vi "single_window_time_all_in_one.vi"(8 "Error In":errorcluster, 9 "Ship data?":bool, 10 "controls":T1={"window duration"=1.0, "width"=5, "crossing level"=0.0, "threshold"=0.25, "Sec"=1.0, "start time"=0.0, "correction thresholds"=[25, 20, 20, 30]} {"start time" format="%#_13g"; "Sec" format="%0.2f"; "threshold" format="%0.2f"; "crossing level" format="%#_13g"; "width" min=3; "window duration" format="%0.2f"}, 11 "waveform in":waveform(dbl)) -> (0 "Error out":errorcluster, 3 "time data cluster":T2 {"variance  of w/a ratio" format="%0.2f"; "sd  of w/a ratio" format="%0.2f"; "mean of w/a ratio" format="%0.2f"})   [LabVIEW 2020]
uses:
  <vilib>/Waveform/WDTOps.llb/WDT Get Waveform Subset DBL.vi
  <vilib>/Analysis/NI_AALBase.lvlib
panel:
  out "XY Graph":T3(graph)
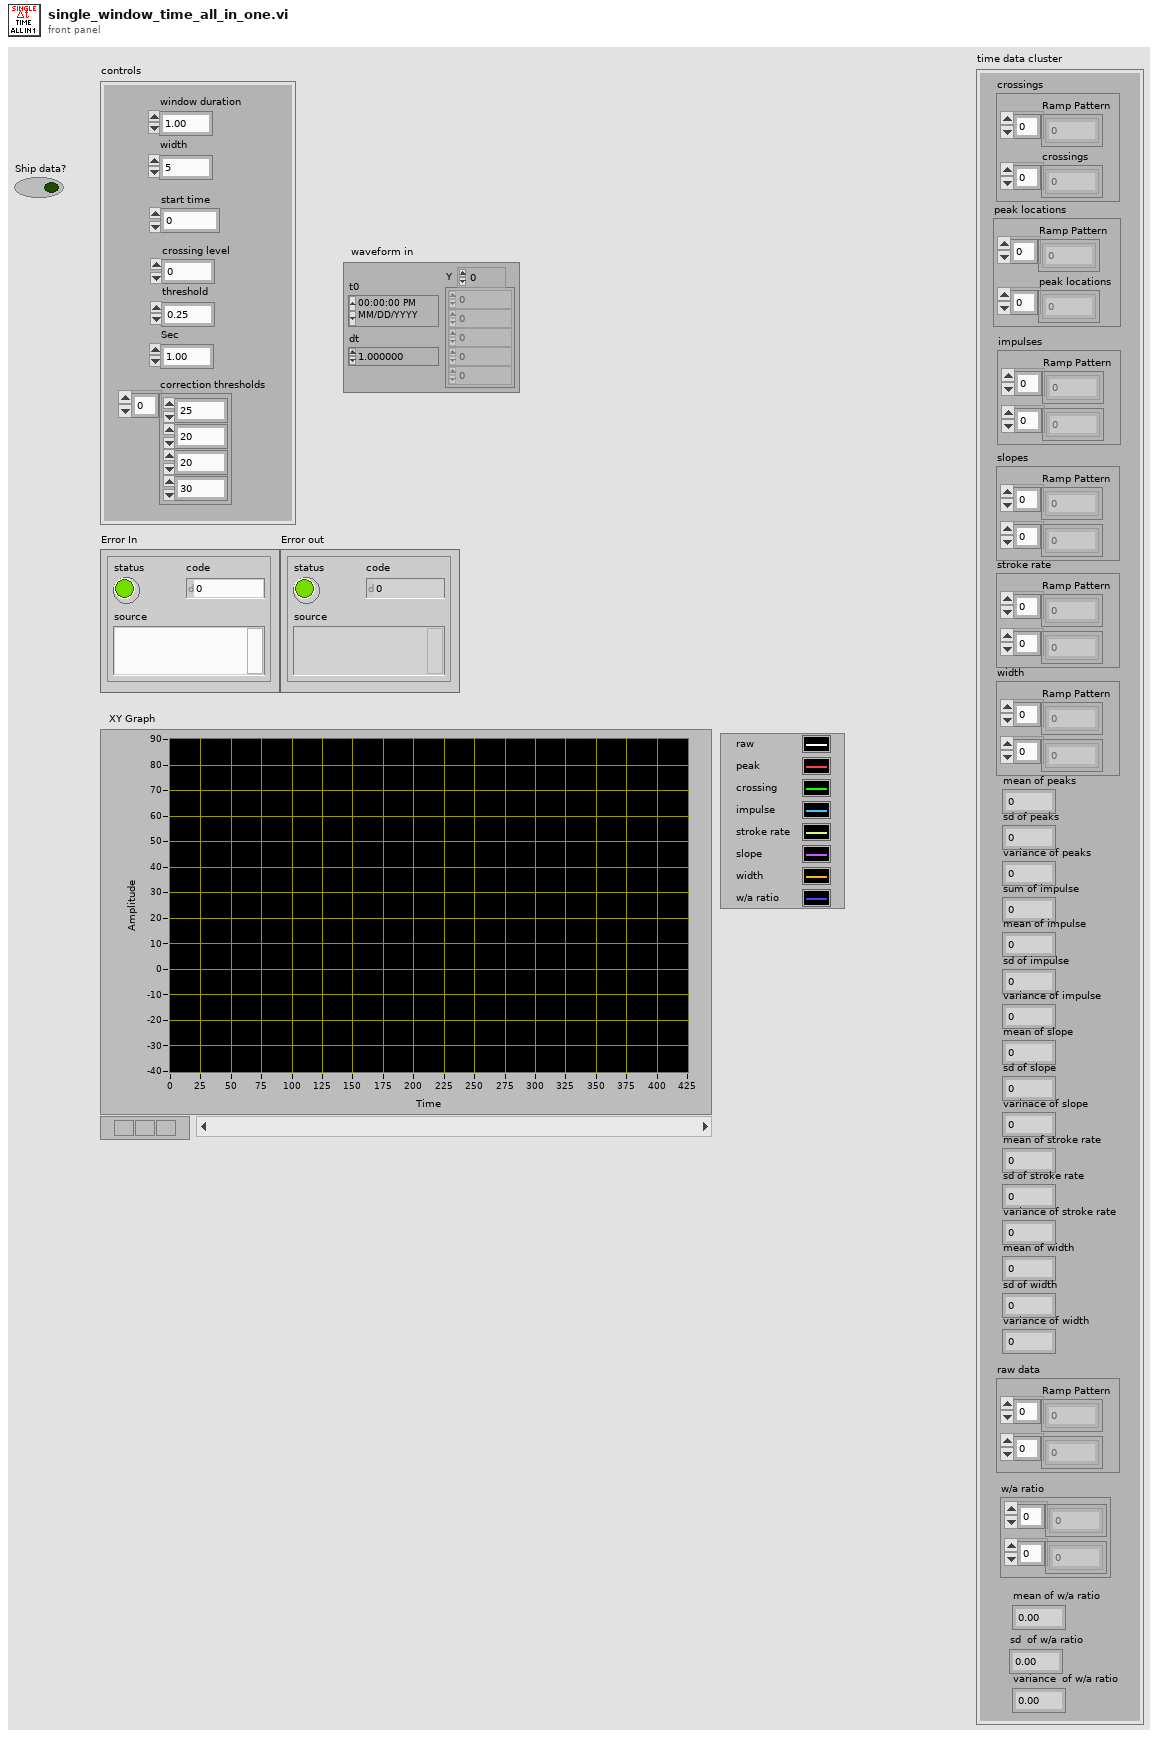
[diagram p1: front panel]
types:
  T1 = cluster{"window duration":dbl, "width":i32, "crossing level":dbl, "threshold":dbl, "Sec":dbl, "start time":dbl, "correction thresholds":i32[]}
  T2 = cluster{"crossings":cluster{"Ramp Pattern":dbl[], "crossings":dbl[]}, "peak locations":cluster{"Ramp Pattern":dbl[], "peak locations":dbl[]}, "impulses":cluster{"Ramp Pattern":dbl[], dbl[]}, "stroke rate":cluster{"Ramp Pattern":dbl[], dbl[]}, "slopes":cluster{"Ramp Pattern":dbl[], dbl[]}, "width":cluster{"Ramp Pattern":dbl[], dbl[]}, "sd of peaks":dbl, "mean of peaks":dbl, "variance of peaks":dbl, "sum of impulse":dbl, "mean of impulse":dbl, "sd of impulse":dbl, "variance of impulse":dbl, "mean of slope":dbl, "sd of slope":dbl, "varinace of slope":dbl, "mean of stroke rate":dbl, "sd of stroke rate":dbl, "variance of stroke rate":dbl, "mean of width":dbl, "sd of width":dbl, "variance of width":dbl, "raw data":cluster{"Ramp Pattern":dbl[], dbl[]}, "w/a ratio":cluster{dbl[], dbl[]}, "mean of w/a ratio":dbl, "sd  of w/a ratio":dbl, "variance  of w/a ratio":dbl}
  T3 = cluster{"Ramp Pattern":dbl[], "peak locations":dbl[]}[]
  T4 = cluster{"Ramp Pattern":dbl[], "peak locations":dbl[]}
  T5 = cluster{"Ramp Pattern":dbl[], "crossings":dbl[]}[]
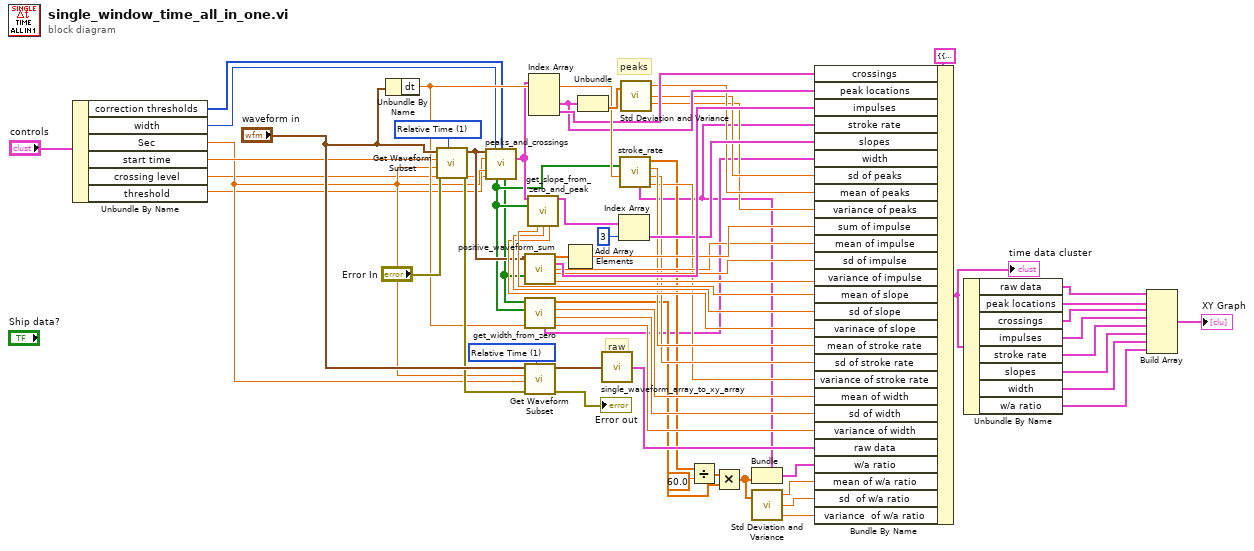
[diagram p0: block diagram]
diagram:
  w61 = u16 1 items=["Samples", "Relative Time"] ("start/duration format")
  w62 = u16 1 items=["Samples", "Relative Time"] ("start/duration format")
  # "raw"
  # "peaks"
  n1 = Unbundle By Name("controls") -> ("correction thresholds"=w15:i32[], "width"=w24:i32, "Sec"=w19:dbl, "start time"=w56:dbl, "crossing level"=w17:dbl, "threshold"=w18:dbl)
  n2 = Unbundle By Name("waveform in") -> ("dt"=w58:dbl)
  n3 = call-poly <vilib>:"Get Waveform Subset.vi"("start/duration format"=w61, "error in (no error)"="Error In", "duration"=w19, "start samples/time"=w56, "waveform in"="waveform in") -> ("error out"=w63:errorcluster, "waveform out"=w23:waveform(dbl))  [unwired: 1 in, 2 out]
  n4 = call "peaks_and_crossings.vi"("waveform"=w23, "width"=w24, "correction thresholds"=w15, "threshold"=w18, "end"=w19, "crossing level"=w17) -> ("all in array"=w22:cluster{dbl[], "Amplitudes":dbl[]}[], "minus-plus crossing?"=w21:bool[], "plus-minus crossing?"=w20:bool[])  [unwired: 3 in, 4 out]
  n5 = call "positive_waveform_sum.vi"("read in data"=w23, "plus-minus"=w20) -> ("impulse"=w57:dbl[], "csapás impulzus"=w44:cluster{"Ramp Pattern":dbl[], dbl[]}, "mean of impulse"=w36:dbl, "sd of impulse"=w35:dbl, "variance of impulse"=w34:dbl)  [unwired: 9 in]
  n6 = call "get_width_from_zero.vi"("dt"=w58, "minus-plus crossing?"=w21, "plus-minus crossing?"=w20) -> ("variance of width"=w25:dbl, "sd of width"=w26:dbl, "mean of width"=w27:dbl, "width"=w11:dbl[], "width graph"=w10:cluster{i32[], dbl[]})  [unwired: 4 in]
  n7 = call-poly <vilib>:"Get Waveform Subset.vi"("start/duration format"=w62, "error in (no error)"=w63, "duration"=w19, "start samples/time"=w19, "waveform in"="waveform in") -> ("error out"=→"Error out":errorcluster, "waveform out"=w66:waveform(dbl))  [unwired: 1 in, 2 out]
  n8 = call "get_slope_from_zero_and_peak.vi"("All in array"=w22, "minus-plus crossing?"=w21) -> ("XY Graph"=w43:cluster{"Array":dbl[], "Amplitudes":dbl[]}[], "slope mean"=w33:dbl, "slope sd"=w32:dbl, "slope variance"=w31:dbl)  [unwired: 8 in, 2 out]
  n9 = Index Array(array=w22) -> (element #2=w45:cluster{dbl[], "Amplitudes":dbl[]}, element #3=w46:cluster{dbl[], "Amplitudes":dbl[]})  [unwired: 3 in, 1 out]
  n10 = Add Array Elements(numeric array=w57) -> (sum=w37:dbl)
  n11 = Unbundle(w45) -> ("Amplitudes"=w59:dbl[])  [unwired: 1 out]
  n12 = call "single_waveform_array_to_xy_array.vi"("waveform in"=w66) -> ("XY out"=w47:cluster{dbl[], "Y":dbl[]})
  n13 = Index Array(array=w43, index=3) -> (element=w41:cluster{"Array":dbl[], "Amplitudes":dbl[]})
  n14 = call "stroke_rate.vi"("dt"=w58, "minus-plus"=w21) -> ("variance of stroke rate"=w28:dbl, "sd  of stroke rate"=w29:dbl, "mean of stroke rate"=w30:dbl, "stroke rate"=w13:dbl[], "stroke rate graph"=w9:cluster{dbl[], dbl[]})  [unwired: 5 in]
  n15 = call <vilib>:"Std Deviation and Variance.vi"("X"=w59) -> ("mean"=w40:dbl, "standard deviation"=w39:dbl, "variance"=w38:dbl)  [unwired: 1 in]
  n16 = Divide(x=w13, y=60.0) -> (x/y=w12:dbl[])
  n17 = Multiply(x=w12, y=w11) -> (x*y=w6:dbl[])
  n18 = Bundle(cluster=w9, w6) -> (w8:cluster{dbl[], dbl[]})  [unwired: 1 in]
  n19 = call <vilib>:"Std Deviation and Variance.vi"("X"=w6) -> ("mean"=w3:dbl, "standard deviation"=w2:dbl, "variance"=w1:dbl)  [unwired: 1 in]
  n20 = Bundle By Name(cluster=T2 {"crossings"={"Ramp Pattern"=[], "crossings"=[]}, "peak locations"={"Ramp Pattern"=[], "peak locations"=[]}, "impulses"={"Ramp Pattern"=[], []}, "stroke rate"={"Ramp Pattern"=[], []}, "slopes"={"Ramp Pattern"=[], []}, "width"={"Ramp Pattern"=[], []}, "sd of peaks"=0.0, "mean of peaks"=0.0, "variance of peaks"=0.0, "sum of impulse"=0.0, "mean of impulse"=0.0, "sd of impulse"=0.0, "variance of impulse"=0.0, "mean of slope"=0.0, "sd of slope"=0.0, "varinace of slope"=0.0, "mean of stroke rate"=0.0, "sd of stroke rate"=0.0, "variance of stroke rate"=0.0, "mean of width"=0.0, "sd of width"=0.0, "variance of width"=0.0, "raw data"={"Ramp Pattern"=[], []}, "w/a ratio"={[], []}, "mean of w/a ratio"=0.0, "sd  of w/a ratio"=0.0, "variance  of w/a ratio"=0.0} ("time data cluster"), "crossings"=w46, "peak locations"=w45, "impulses"=w44, "stroke rate"=w9, "slopes"=w41, "width"=w10, "sd of peaks"=w39, "mean of peaks"=w40, "variance of peaks"=w38, "sum of impulse"=w37, "mean of impulse"=w36, "sd of impulse"=w35, "variance of impulse"=w34, "mean of slope"=w33, "sd of slope"=w32, "varinace of slope"=w31, "mean of stroke rate"=w30, "sd of stroke rate"=w29, "variance of stroke rate"=w28, "mean of width"=w27, "sd of width"=w26, "variance of width"=w25, "raw data"=w47, "w/a ratio"=w8, "mean of w/a ratio"=w3, "sd  of w/a ratio"=w2, "variance  of w/a ratio"=w1) -> (w4:T2)
  "time data cluster" <- w4
  n21 = Unbundle By Name(w4) -> ("raw data"=w48:cluster{"Ramp Pattern":dbl[], dbl[]}, "peak locations"=w55:T4, "crossings"=w54:cluster{"Ramp Pattern":dbl[], "crossings":dbl[]}, "impulses"=w53:cluster{"Ramp Pattern":dbl[], dbl[]}, "stroke rate"=w52:cluster{"Ramp Pattern":dbl[], dbl[]}, "slopes"=w51:cluster{"Ramp Pattern":dbl[], dbl[]}, "width"=w50:cluster{"Ramp Pattern":dbl[], dbl[]}, "w/a ratio"=w7:cluster{dbl[], dbl[]})
  n22 = Build Array(w48, w55, w54, w53, w52, w51, w50, w7) -> (→"XY Graph":T5)
